vi "set radix.vi"(8 "error in (no error)":errorcluster, 10 "Radix":T1, 11 "Digital in":refnum<vi>) -> (0 "error out":errorcluster)   [LabVIEW 2021, in "Modbus Master System Explorer.lvlib"]
uses:
  Modbus Master System Explorer.lvlib
  Radix.ctl
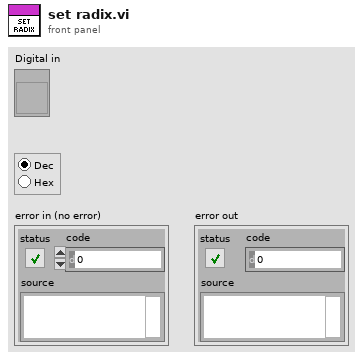
[diagram p1: front panel]
types:
  T1 = typedef "Modbus Master System Explorer.lvlib/Radix.ctl" = enum32{"Decimal", "Hexidecimal"}
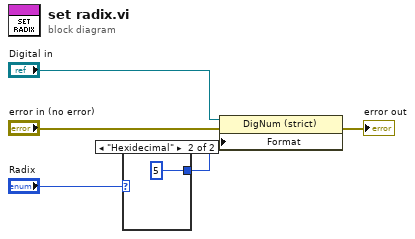
[diagram p0: block diagram]
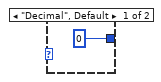
[diagram p2: hidden frame]
diagram:
  n1 = case shown="\"Hexidecimal\"" "Radix" {
    tunnel: [u8 0 u8 5] -> w5
    frame "Decimal", Default {
    }
    frame "Hexidecimal" {
    }
  }
  n2 = property on="Property Node" class="DigNum (strict)"(reference="Digital in", error in="error in (no error)", "Format"=w5) -> (error out=→"error out":errorcluster)  [unwired: 1 out]
